vi "Oluwatofunmi_Sodimu_Hodgkin-Huxley model.vi"() -> ()   [LabVIEW 2020]
uses:
  <vilib>/Simulation/Scripting/Companion Diagram/SimConfigNode/SimParams.ctl
  <vilib>/Simulation/Scripting/Companion Diagram/SimConfigNode/_simSolvers.ctl
  <vilib>/Simulation/Implementation/Shared/SIMSCR Execution Mode.ctl
  <vilib>/Simulation/Param Hierarchy/Typedefs/SIMPH Param Control Actions.ctl
  <vilib>/Simulation/Implementation/Shared/SIM limit type.ctl
  <vilib>/Simulation/Implementation/Shared/NILVSim_ParamChanged.vi
  <vilib>/Simulation/Implementation/Shared/NILVSIM_BeginStep.vi
  <vilib>/Simulation/DataSources/Implementation/NILVSim Pulse Generator.llb/SIM Pulse Generator (scalar).vi
  <vilib>/Simulation/SignalDisplay/Implementation/NILVSim Time Waveform.llb/SIM Time Waveform (scalar).vi
  <vilib>/Simulation/ContinuousLinear/Implementation/NILVSim Integrator new.llb/SIM Integrator distributor (scalar).vi
  <vilib>/Simulation/Nonlinear/Implementation/NILVSim Saturation.llb/SIM Saturation (scalar).vi
  <vilib>/Simulation/ContinuousLinear/Implementation/NILVSim Integrator new.llb/SIM Integrator collector (scalar).vi
  <vilib>/Simulation/SignalDisplay/Implementation/NILVSim Time Waveform.llb/SIM Time Waveform (vector).vi
  <vilib>/Simulation/Implementation/Shared/NILVSim_Manager.vi
  <vilib>/Utility/error.llb/Clear Errors.vi
  <vilib>/Simulation/Implementation/Shared/NILVSim_FinalizeModel.vi
  <vilib>/Simulation/Implementation/Shared/SIM Unbundle Sim Info.vi
  <vilib>/Simulation/Implementation/Shared/NILVSim_Initialize.vi
  <vilib>/Simulation/Utility/Implementation/NILVSim Get Time and IsAcceptedStep.vi
  <vilib>/Simulation/Implementation/Shared/SIMSH Read Queue.vi
  <vilib>/Simulation/Implementation/Shared/NILVSim_GetModelError.vi
  <vilib>/Simulation/Implementation/Shared/SIM Bundle Sim Info.vi
  <vilib>/Simulation/Scripting/Companion Diagram/SimConfigNode/SimDog.xnode
  <vilib>/Simulation/Model Libraries/PID/SIM PID (Parallel).vi
  <vilib>/Simulation/Model Libraries/PID/SIM PID.vi
  <vilib>/Simulation/Implementation/XNodeFramework/SimXNode/SimX.xnode
  <vilib>/Simulation/ContinuousLinear/Implementation/NILVSim Integrator new.llb/SIM Integrator (scalar).vi
  <vilib>/Simulation/Implementation/Shared/NI_SIM_Implementation.lvlib
panel:
  in  "Derivative Gain":dbl=1.0
  in  "Integral Gain":dbl
  in  "Proportional Gain":dbl
  out "Vo":dbl format="%#_13g"
  out "Steady State current":dbl format="%#_13g"
  out "Reference Voltage":waveform(dbl)(graph)={"t0"=timestamp(25 s since 1904-01-01), "dt"=1.0, "Y"=[100.0]}
  out "Error signal":waveform(dbl)(graph)={"t0"=timestamp(25 s since 1904-01-01), "dt"=1.0, "Y"=[0.11092075631839293]}
  in  "Voltage\nAmplitude":dbl=100.0
  in  "Voltage \nON TIME (msec)":dbl=10.0 format="%#_13g"
  in  "Voltage\nOFF TIME(msec)":dbl format="%#_13g"
  in  "Saturation \nlower limit":dbl=-6000.0
  in  "Saturation\nUpper limit":dbl=6000.0
  in  "Controller":bool=TRUE
  in  "Step Size (s)":dbl=0.001
  in  "ODE Solver":T1(ring)=enum."Runge-Kutta 4"
  in  "Final Simulation Time (ms)":dbl=25.0
  out "Membrane\nvoltage(shifted)":waveform(dbl)(graph)={"t0"=timestamp(25 s since 1904-01-01), "dt"=1.0, "Y"=[99.8890792436816]}
  in  "OFF TIME(msec)":dbl
  in  "ON TIME(msec)":dbl=10.0
  out "Conductances":waveform(dbl)[](graph)=[{"t0"=timestamp(25 s since 1904-01-01), "dt"=1.0, "Y"=[0.05668572584751632]}, {"t0"=timestamp(25 s since 1904-01-01), "dt"=1.0, "Y"=[30.781462329577824]}]
  out "Applied Current":waveform(dbl)(graph)={"t0"=timestamp(25 s since 1904-01-01), "dt"=1.0, "Y"=[3470.066355678789]}
  out "Gating Variables":waveform(dbl)[](graph)=[{"t0"=timestamp(25 s since 1904-01-01), "dt"=1.0, "Y"=[0.997927299463547]}, {"t0"=timestamp(25 s since 1904-01-01), "dt"=1.0, "Y"=[0.9616049423275413]}, {"t0"=timestamp(25 s since 1904-01-01), "dt"=1.0, "Y"=[0.00047533058062492964]}]
  in  "Membrane\nCapacitance(Cm)":dbl=1.0
  in  "Leakage \nConductance (gL)":dbl=0.3
  in  "Shifted equilibrium\npotential for leakage (Vl)":dbl=10.6
  in  "Shifted equilibrium\npotential for Na (Vna)":dbl=115.0
  in  "Maximal Na\nconductance (gNa)":dbl=120.0
  in  "Applied current (Iapp)":dbl=5.0
  in  "Shifted equilibrium\npotential for k (Vk)":dbl=-12.0
  in  "Maximal K \nconductance (gk)":dbl=36.0 format="%#_13g"
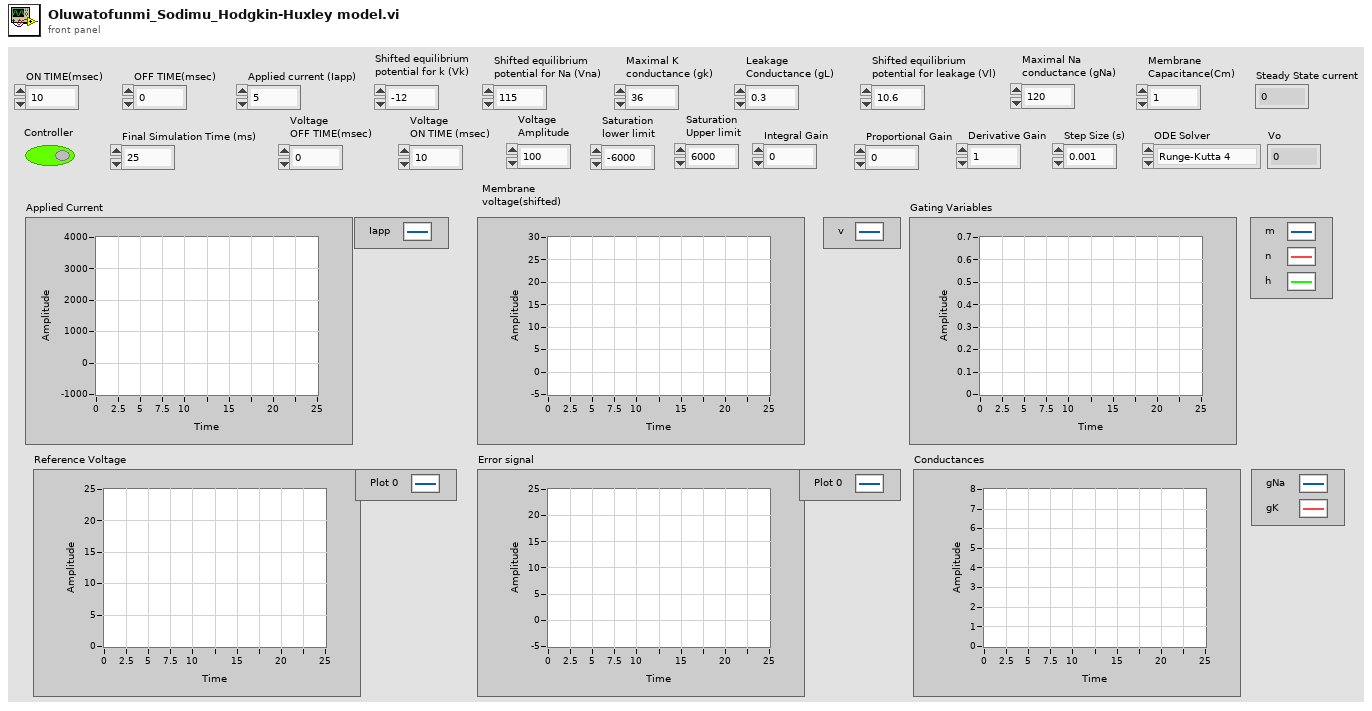
[diagram p1: front panel]
types:
  T1 = enum16{"Runge-Kutta 1 (Euler)", "Runge-Kutta 2", "Runge-Kutta 3", "Runge-Kutta 4", "Runge-Kutta 23 (variable)", "Runge-Kutta 45 (variable)", "BDF (variable)", "Adams-Moulton (variable)", "Rosenbrock (variable)", "Discrete States Only", "SDIRK 4 (variable)", "Radau 5 (variable)", "Radau 9 (variable)", "Radau 13 (variable)", "Radau [Variable Order] (variable)", "Gear's Method (variable)"}
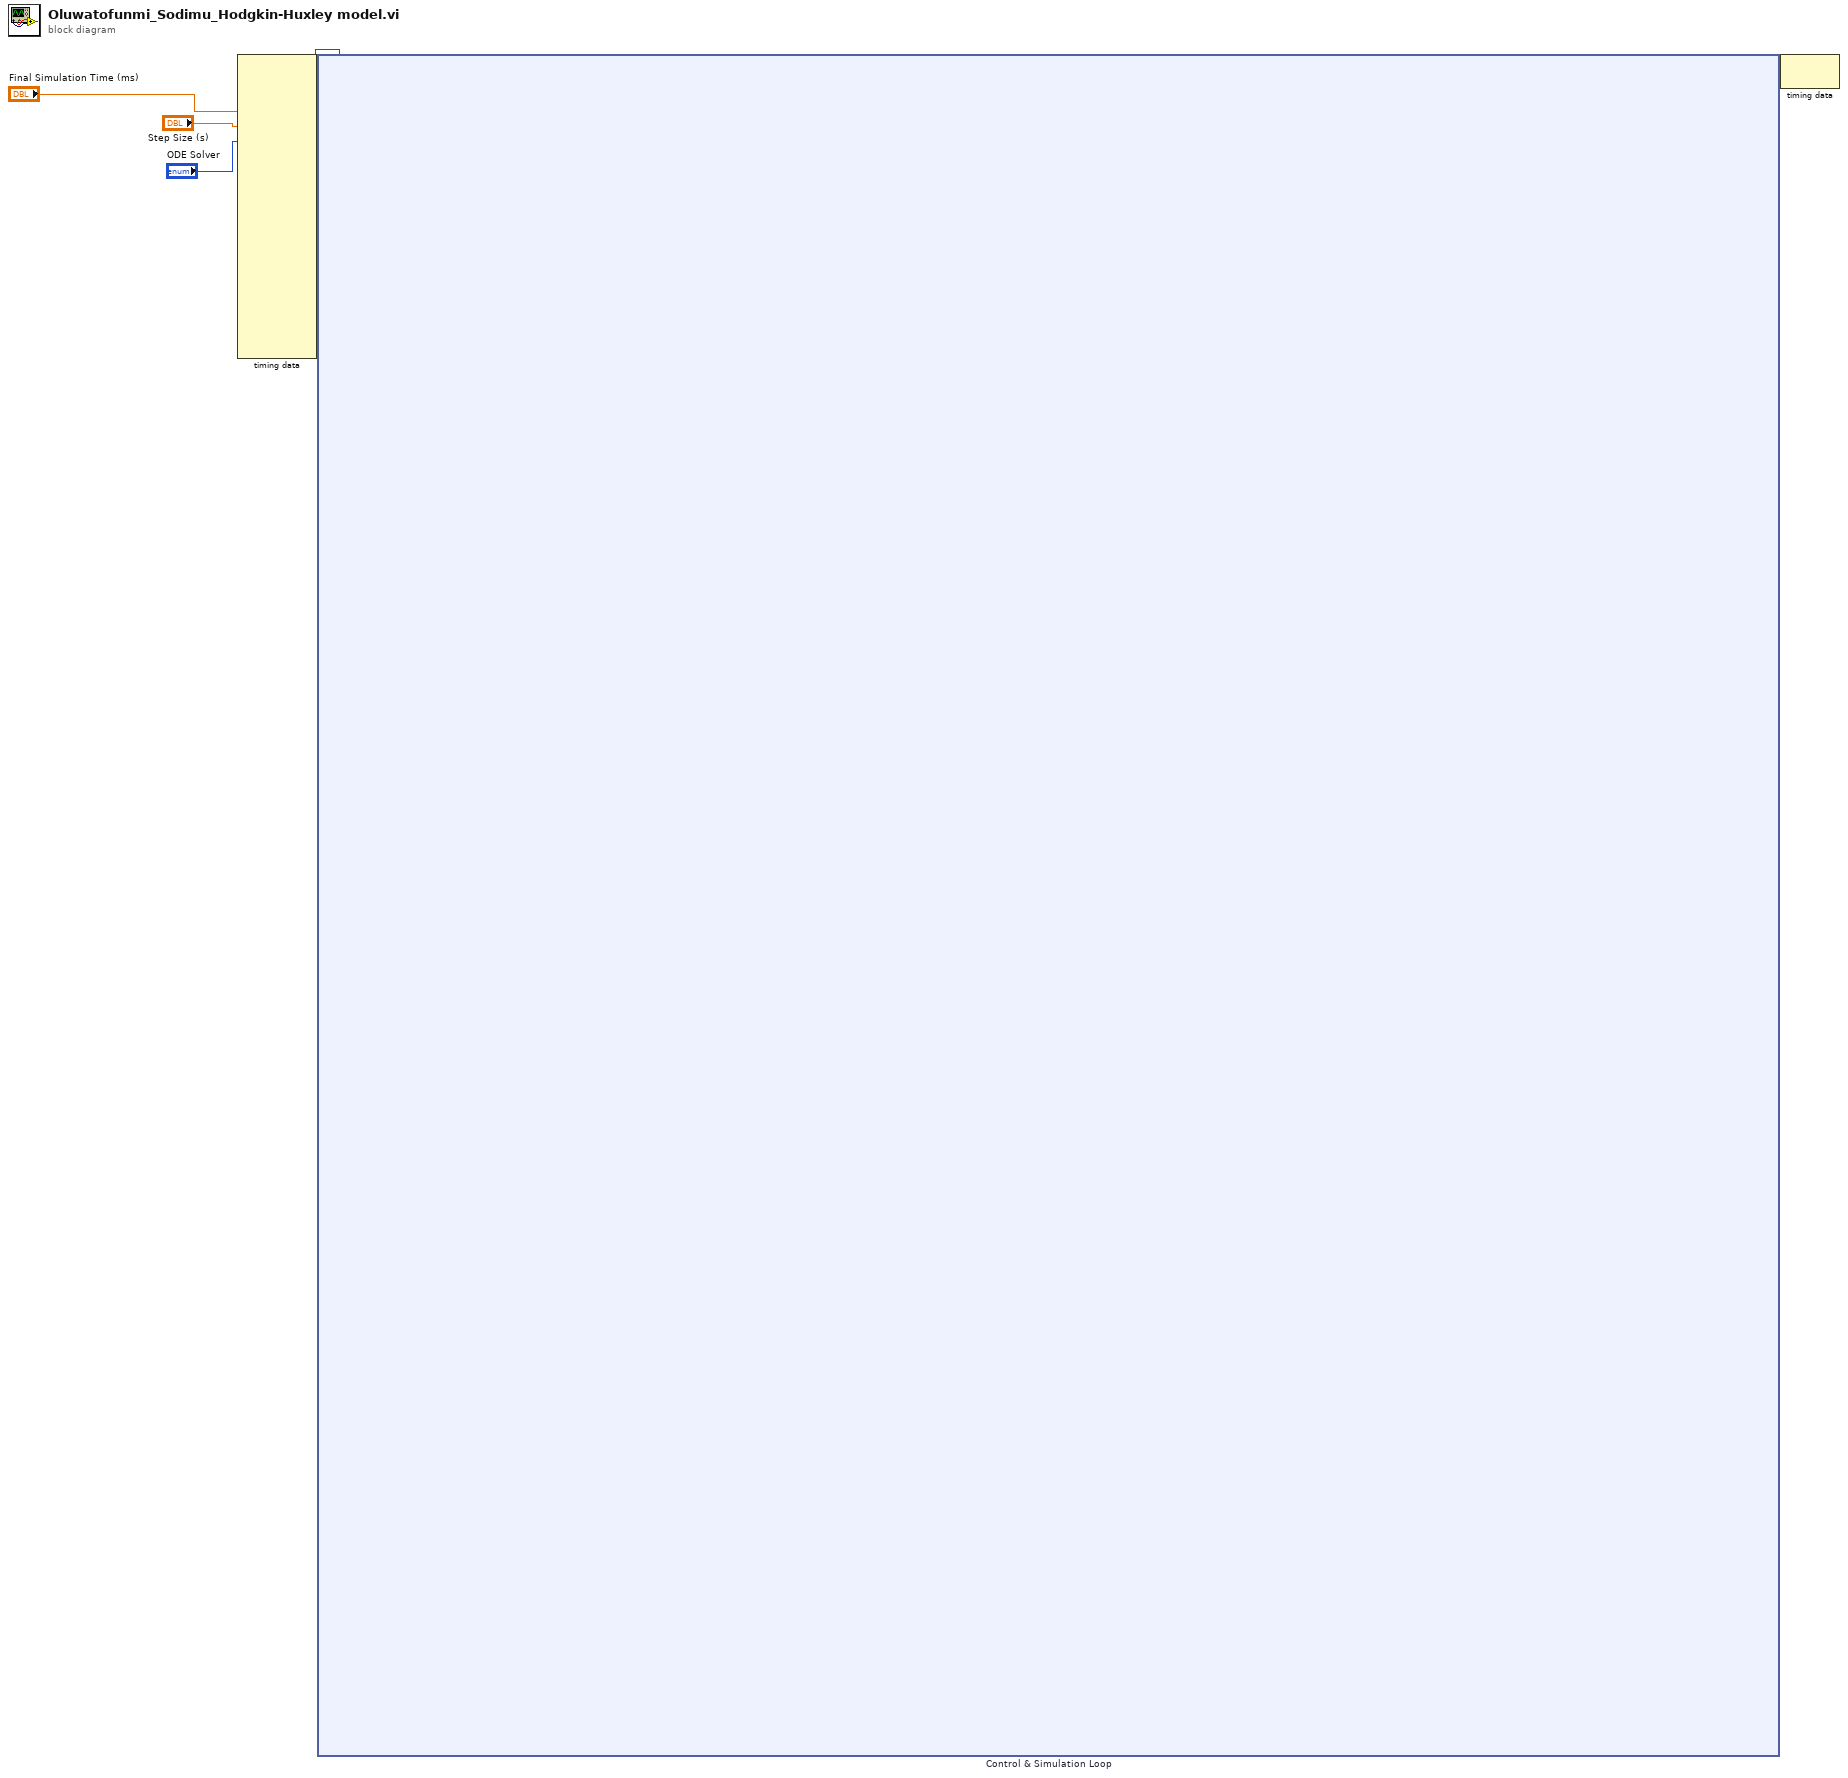
[diagram p0: block diagram]
diagram:
  n1 = node-c288("Final Simulation Time (ms)", "Step Size (s)", "ODE Solver") -> (w5:variant)  [unwired: 16 in]
  n2 = node-c254 "Control & Simulation Loop"(w5) -> (w4:variant)
  n3 = node-c288(w4) -> ()  [unwired: 1 out]
